vi "SeCrTs - DD obtain Queue.vi"(8 "error in":errorcluster) -> (0 "error out":errorcluster, 2 "AI_V_Data P\nAI_C_Data P\nAO_Data P\nDO_Data P\nACC_Data P\nTC Data P\nDrive_A_C \nDrive_A_D\nAI_C_Data S\nDO_Data S":refnum<queue>[](array[refnum]), 3 "DI P\nDI S":refnum<queue>[](array[refnum]))   [LabVIEW 2022 SP3]
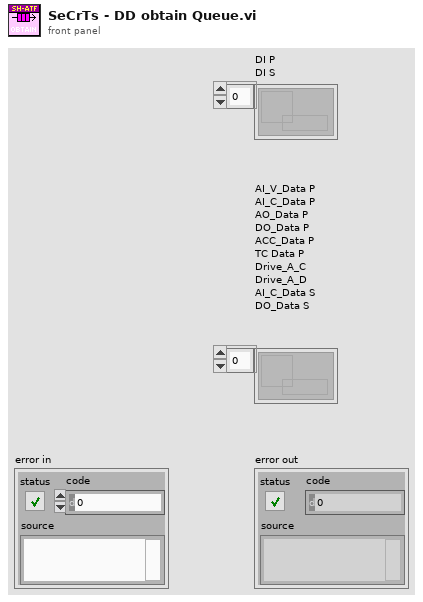
[diagram p1: front panel]
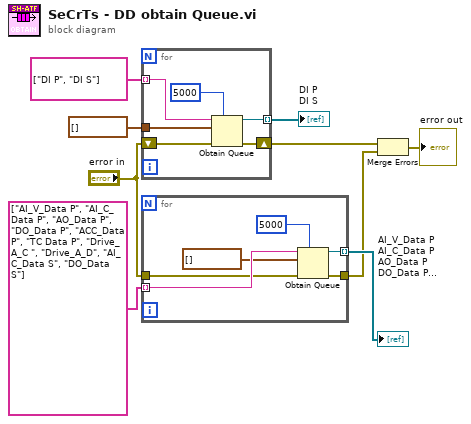
[diagram p0: block diagram]
diagram:
  n1 = for {
    tunnel: digitalwaveform[] [] ("DI_Data") -> [w15]
    tunnel: string[] ["DI P", "DI S"] ("name (unnamed)") -> [w14] mode=indexing
    tunnel: [w11] -> w1 mode=indexing
    shift-right: [w10] -> w2
    shift-left: "error in" -> [w12]
    n2 = Obtain Queue(max queue size (-1, unlimited)=5000, name (unnamed)=w14, element data type=w15, error in (no error)=w12) -> (queue out=w11:refnum<queue>, error out=w10:errorcluster)  [unwired: 1 in, 1 out]
  }
  "DI P\nDI S" <- w1
  n3 = for {
    tunnel: string[] ["AI_V_Data P", "AI_C_Data P", "AO_Data P", "DO_Data P", "ACC_Data P", "TC Data P", "Drive_A_C ", "Drive_A_D", "AI_C_Data S", "DO_Data S"] ("Array") -> [w21] mode=indexing
    tunnel: "error in" -> [w19]
    tunnel: [w18] -> w5 mode=indexing
    tunnel: [w17] -> w4
    n4 = Obtain Queue(max queue size (-1, unlimited)=5000, name (unnamed)=w21, element data type=waveform(dbl)[] [] ("AI_V_Data"), error in (no error)=w19) -> (queue out=w18:refnum<queue>, error out=w17:errorcluster)  [unwired: 1 in, 1 out]
  }
  "AI_V_Data P\nAI_C_Data P\nAO_Data P\nDO_Data P\nACC_Data P\nTC Data P\nDrive_A_C \nDrive_A_D\nAI_C_Data S\nDO_Data S" <- w5
  n5 = Merge Errors(w2, w4) -> (→"error out":errorcluster)
